vi "tache.vi"() -> ()   [LabVIEW 2024]
panel:
  in  "Name":string
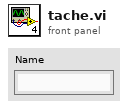
[diagram p1: front panel]
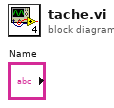
[diagram p0: block diagram]
diagram:
